vi "Framework Listener Sobot.vi"() -> ()   [LabVIEW 2017]
uses:
  TypeDefinitions/TCP Cluster.ctl
  TypeDefinitions/TCP Commands.ctl
  TypeDefinitions/Sobot Driving Data.ctl
  <vilib>/Utility/inputDevices.llb/closeJoystick.vi
  <vilib>/Instr/_visa.llb/VISA Configure Serial Port (Instr).vi
panel:
  out "value":T1
  out "Driving Data":u8[](array[numeric])
  in  "stop 2":bool
  in  "device index":i32
  in  "Manuelles Fahren (Joystick)":bool
  in  "VISA resource name":refnum<visa-resource-name>
  out "Send":T2={"Datatype"=enum."Message", "String"="Send to sobot"}
  out "Receive":T2={"Datatype"=enum."Message", "String"="Send to sobot"}
  in  "Button 2":bool
  in  "stop":bool
  in  "Button 1":bool
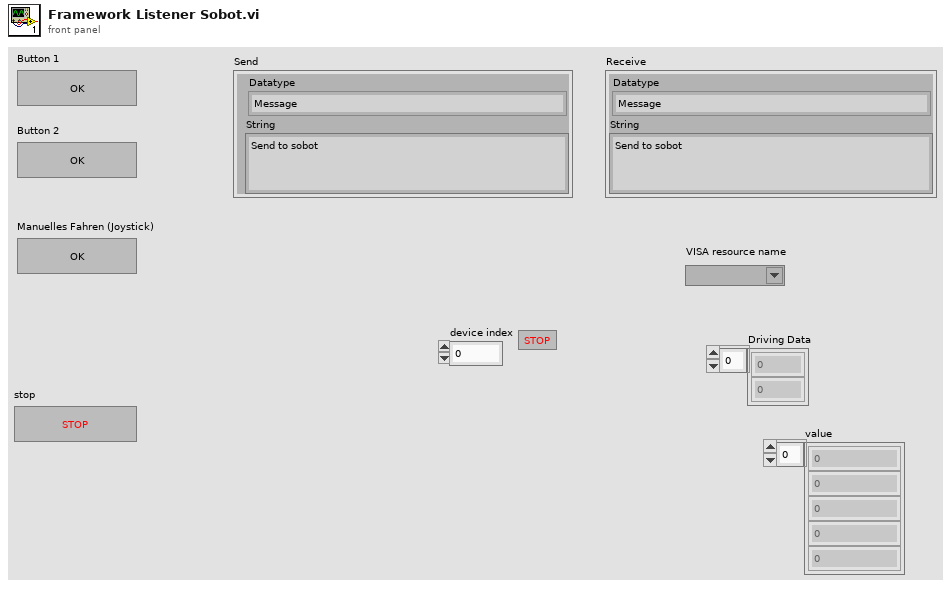
[diagram p1: front panel]
types:
  T1 = typedef "Sobot Driving Data.ctl" = u8[]
  T2 = typedef "TCP Cluster.ctl" = cluster{"Datatype":T3, "String":string}
  T3 = typedef "TCP Commands.ctl" = enum16{"Message", "sobotManualDrive", "Stop", "Command"}
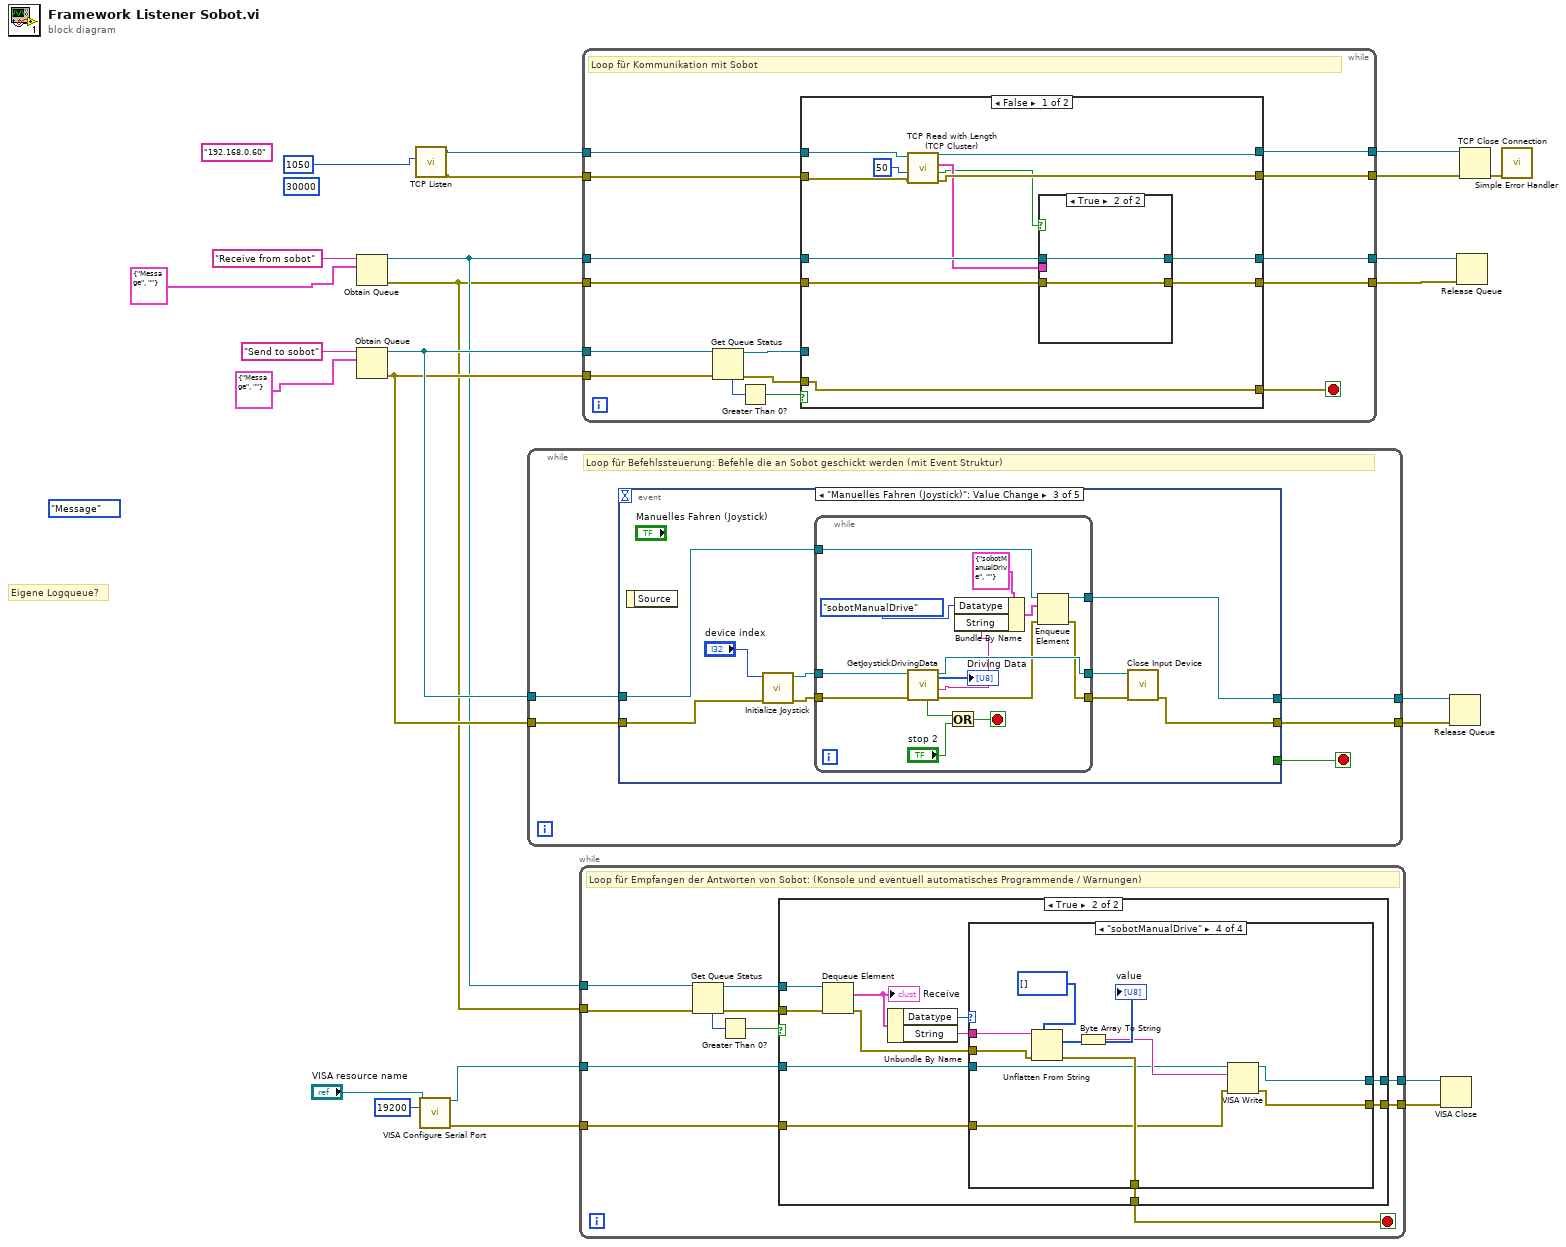
[diagram p0: block diagram]
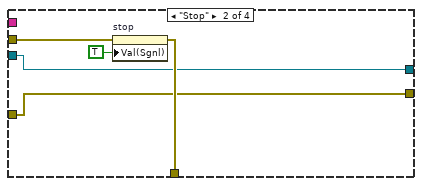
[diagram p4: hidden frame]
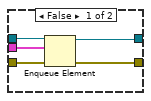
[diagram p6: hidden frame]
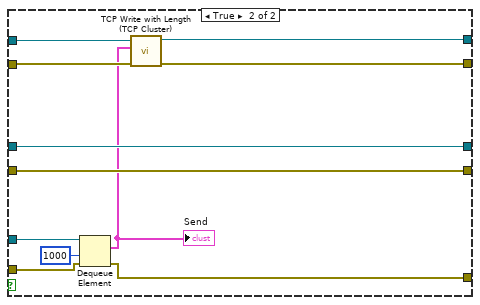
[diagram p7: hidden frame]
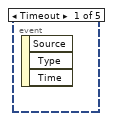
[diagram p8: hidden frame]
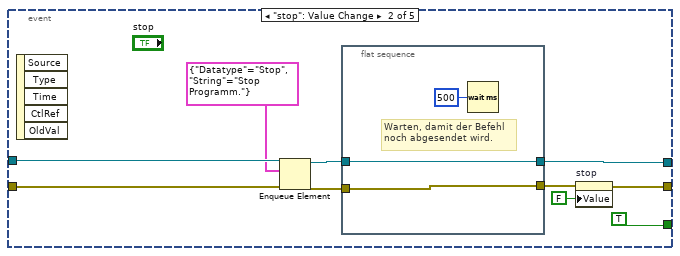
[diagram p9: hidden frame]
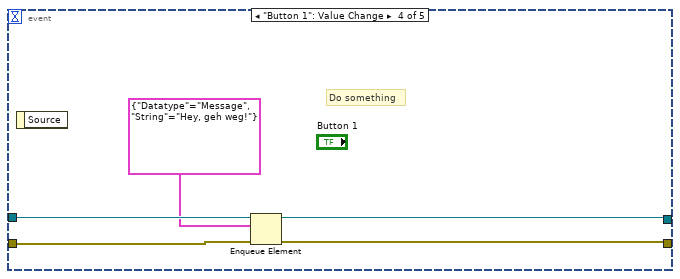
[diagram p10: hidden frame]
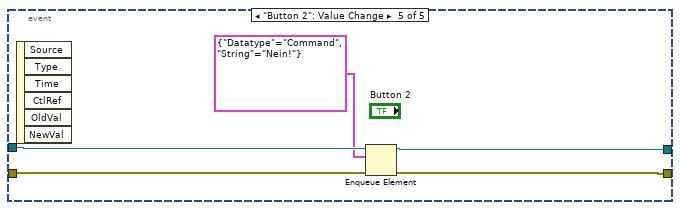
[diagram p11: hidden frame]
diagram:
  (unwired) TCP_Commands."Message"
  (unwired) 30000 ("timeout ms (60000)")
  (unwired) "192.168.0.60" ("address")
  # "Eigene Logqueue?"
  n1 = Obtain Queue(name (unnamed)="Receive from sobot", element data type=T2 {"Datatype"=enum."Message", "String"=""}) -> (queue out=w15:refnum<queue>, error out=w14:errorcluster)  [unwired: 3 in, 1 out]
  n2 = Obtain Queue(name (unnamed)="Send to sobot", element data type=T2 {"Datatype"=enum."Message", "String"=""}) -> (queue out=w23:refnum<queue>, error out=w20:errorcluster)  [unwired: 3 in, 1 out]
  n3 = call <vilib>:"TCP Listen.vi"("port"=u16 1050 ("remote port or service name")) -> ("error out"=w2:errorcluster, "connection ID"=w3:refnum<k5>)  [unwired: 6 in, 3 out]
  n4 = call-poly "VISA Configure Serial Port"("VISA resource name"="VISA resource name", "baud rate (9600)"=u32 19200) -> ("VISA resource name out"=w5:refnum<visa-resource-name>, "error out"=w4:errorcluster)  [unwired: 12 in]
  n5 = while {
    tunnel: w23 -> [w28]
    tunnel: [w27] -> w22
    tunnel: [w26] -> w21
    tunnel: w20 -> [w25]
    stop <- w29 stop-if-true
    # "Loop für Befehlssteuerung: Befehle die an Sobot geschickt werden (mit Event Struktur)"
    n6 = event shown="[2] \"Manuelles Fahren (Joystick)\": Value Change" {
      selector: _ -> [_ _ _ _ _]
      dyn-events: _ -> [_ _ _ _ _]
      timeout: _ -> [_ _ _ _ _]
      tunnel: [_ TRUE _ _ _] -> w29
      tunnel: w28 -> [_ w38 w44 w71 w76]
      tunnel: [_ w34 w43 w68 w75] -> w27
      tunnel: [_ w31 w45 w69 w74] -> w26
      tunnel: w25 -> [_ w37 w46 w70 w73]
      event Timeout {
        n7 = event-data() -> ()  [unwired: 1 in, 3 out]
      }
      event "stop": Value Change {
        n8 = event-data() -> ()  [unwired: 1 in, 5 out]
        n9 = Enqueue Element(queue=w38, element=T2 {"Datatype"=enum."Stop", "String"="Stop Programm."}, error in (no error)=w37) -> (queue out=w35:refnum<queue>, error out=w33:errorcluster)  [unwired: 1 in, 1 out]
        n10 = flat-sequence {
          tunnel: w35 -> [w42]
          tunnel: [w42] -> w34
          tunnel: [w40] -> w32
          tunnel: w33 -> [w40]
          frame #0 {
            # "Warten, damit der Befehl\nnoch abgesendet wird."
            n11 = Wait (ms)(milliseconds to wait=u32 500) -> ()  [unwired: 1 out]
          }
        }
        n12 = property on="stop" class="Bool (strict)"(error in=w32, "Value"=FALSE ("stop")) -> (error out=w31:errorcluster)  [unwired: 1 in, 1 out]
      }
      event "Manuelles Fahren (Joystick)": Value Change {
        n13 = event-data() -> ()  [unwired: 1 in, 1 out]
        n14 = call <vilib>:"Initialize Joystick.vi"("error in (no error)"=w46, "device index"="device index") -> ("error out"=w50:errorcluster, "device ID"=w51:refnum<k1>)  [unwired: 8 in]
        n15 = while {
          tunnel: w51 -> [w66]
          tunnel: w50 -> [w65]
          tunnel: [w64] -> w48
          tunnel: [w52] -> w47
          tunnel: w44 -> [w55]
          tunnel: [w54] -> w43
          stop <- w61 stop-if-true
          n16 = call "GetJoystickDrivingData.vi"("error in (no error)"=w65, "Refnum in"=w66) -> ("error out"=w53:errorcluster, "data string"=w58:string, "Refnum out"=w64:refnum<k1>, "Boolean"=w62:bool, "Array"=→"Driving Data":u8[])  [unwired: 4 in, 1 out]
          n17 = Or(x=w62, y="stop 2") -> (x .or. y?=w61:bool)
          n18 = Bundle By Name(cluster=T2 {"Datatype"=enum."sobotManualDrive", "String"=""}, "Datatype"=TCP_Commands."sobotManualDrive", "String"=w58) -> (w56:T2)
          n19 = Enqueue Element(queue=w55, element=w56, error in (no error)=w53) -> (queue out=w54:refnum<queue>, error out=w52:errorcluster)  [unwired: 1 in, 1 out]
        }
        n20 = call-poly <vilib>:"Close Input Device.vi"("error in (no error)"=w47, "device ID"=w48) -> ("error out"=w45:errorcluster)  [unwired: 8 in]
      }
      event "Button 1": Value Change {
        # "Do something"
        n21 = event-data() -> ()  [unwired: 1 in, 1 out]
        n22 = Enqueue Element(queue=w71, element=T2 {"Datatype"=enum."Message", "String"="Hey, geh weg!"}, error in (no error)=w70) -> (queue out=w68:refnum<queue>, error out=w69:errorcluster)  [unwired: 1 in, 1 out]
      }
      event "Button 2": Value Change {
        n23 = event-data() -> ()  [unwired: 1 in, 6 out]
        n24 = Enqueue Element(queue=w76, element=T2 {"Datatype"=enum."Command", "String"="Nein!"}, error in (no error)=w73) -> (queue out=w75:refnum<queue>, error out=w74:errorcluster)  [unwired: 1 in, 1 out]
      }
    }
  }
  n25 = while {
    tunnel: w15 -> [w86]
    tunnel: w14 -> [w85]
    tunnel: [w80] -> w9
    tunnel: [w79] -> w8
    tunnel: w5 -> [w78]
    tunnel: w4 -> [w77]
    stop <- w81 stop-if-true
    # "Loop für Empfangen der Antworten von Sobot: (Konsole und eventuell automatisches Programmende / Warnungen)"
    n26 = Get Queue Status(queue=w86, error in (no error)=w85) -> (queue out=w83:refnum<queue>, error out=w82:errorcluster, # elements in queue=w87:i32)  [unwired: 1 in, 5 out]
    n27 = Greater Than 0?(x=w87) -> (x > 0?=w84:bool)
    n28 = case shown="True" w84 {
      tunnel: w83 -> [_ w101]
      tunnel: w82 -> [w90 w100]
      tunnel: [w90 w96] -> w81
      tunnel: [w88 w94] -> w80
      tunnel: [w89 w93] -> w79
      tunnel: w78 -> [w89 w92]
      tunnel: w77 -> [w88 w91]
      frame False {
      }
      frame True {
        n29 = Dequeue Element(queue=w101, error in (no error)=w100) -> (element=w99:T2, error out=w97:errorcluster)  [unwired: 1 in, 2 out]
        "Receive" <- w99
        n30 = Unbundle By Name(w99) -> ("Datatype"=w98:T3, "String"=w95:string)
        n31 = case shown="\"sobotManualDrive\"" w98 {
          tunnel: w97 -> [w104 w108 w112 w120]
          tunnel: [w104 w107 w112 w119] -> w96
          tunnel: w95 -> [_ _ _ w122]
          tunnel: [w102 w105 w110 w116] -> w94
          tunnel: [w103 w106 w111 w115] -> w93
          tunnel: w92 -> [w103 w106 w111 w114]
          tunnel: w91 -> [w102 w105 w110 w113]
          frame "Message", Default {
          }
          frame "Stop" {
            n32 = property on="stop" class="Bool (strict)"(error in=w108, "Val(Sgnl)"=TRUE ("Value (Signaling)")) -> (error out=w107:errorcluster)  [unwired: 1 in, 1 out]
          }
          frame "Command" {
          }
          frame "sobotManualDrive" {
            n33 = Unflatten From String(type=T1 [] ("Sobot Driving Data"), binary string=w122, error in (no error)=w120) -> (value=w118:T1, error out=w119:errorcluster)  [unwired: 2 in, 1 out]
            "value" <- w118
            n34 = Byte Array To String(unsigned byte array=w118) -> (string=w117:string)
            n35 = VISA Write(VISA resource name=w114, write buffer=w117, error in (no error)=w113) -> (VISA resource name out=w115:refnum<visa-resource-name>, error out=w116:errorcluster)  [unwired: 1 out]
          }
        }
      }
    }
  }
  n36 = while {
    tunnel: w23 -> [w136]
    tunnel: w20 -> [w134]
    tunnel: w3 -> [w130]
    tunnel: w2 -> [w129]
    tunnel: [w128] -> w18
    tunnel: [w127] -> w17
    tunnel: w15 -> [w126]
    tunnel: w14 -> [w125]
    tunnel: [w124] -> w12
    tunnel: [w123] -> w13
    stop <- w137 stop-if-true
    # "Loop für Kommunikation mit Sobot"
    n37 = Get Queue Status(queue=w136, error in (no error)=w134) -> (queue out=w135:refnum<queue>, error out=w133:errorcluster, # elements in queue=w132:i32)  [unwired: 1 in, 5 out]
    n38 = Greater Than 0?(x=w132) -> (x > 0?=w131:bool)
    n39 = case shown="False" w131 {
      tunnel: [w149 w167] -> w137
      tunnel: w135 -> [_ w165]
      tunnel: w133 -> [w149 w164]
      tunnel: w130 -> [w144 w161]
      tunnel: w129 -> [w143 w160]
      tunnel: [w141 w159] -> w127
      tunnel: [w140 w158] -> w128
      tunnel: w126 -> [w148 w163]
      tunnel: w125 -> [w147 w162]
      tunnel: [w146 w163] -> w123
      tunnel: [w145 w162] -> w124
      frame False {
        n40 = call "TCP Read with Length (TCP Cluster).vi"("error in (no error)"=w143, "Timeout"=50, "connection ID"=w144) -> ("error out"=w141:errorcluster, "Timeout?"=w138:bool, "TCP Cluster"=w139:T2, "connection ID out"=w140:refnum<k5>)  [unwired: 5 in]
        n41 = case shown="True" w138 {
          tunnel: w148 -> [w154 w156]
          tunnel: w147 -> [w153 w155]
          tunnel: w139 -> [w152 _]
          tunnel: [w151 w156] -> w146
          tunnel: [w150 w155] -> w145
          frame False {
            n42 = Enqueue Element(queue=w154, element=w152, error in (no error)=w153) -> (queue out=w151:refnum<queue>, error out=w150:errorcluster)  [unwired: 1 in, 1 out]
          }
          frame True {
          }
        }
      }
      frame True {
        n43 = Dequeue Element(queue=w165, timeout in ms (-1)=1000, error in (no error)=w164) -> (element=w157:T2, error out=w167:errorcluster)  [unwired: 2 out]
        "Send" <- w157
        n44 = call "TCP Write with Length (TCP Cluster).vi"("error in (no error)"=w160, 10:w157, "connection ID"=w161) -> ("error out"=w159:errorcluster, "connection ID out"=w158:refnum<k5>)  [unwired: 7 in]
      }
    }
  }
  n45 = VISA Close(VISA resource name=w8, error in (no error)=w9) -> ()  [unwired: 1 out]
  n46 = Release Queue(queue=w22, error in (no error)=w21) -> ()  [unwired: 1 in, 3 out]
  n47 = Release Queue(queue=w13, error in (no error)=w12) -> ()  [unwired: 1 in, 3 out]
  n48 = TCP Close Connection(connection ID=w18, error in (no error)=w17) -> (error out=w19:errorcluster)  [unwired: 1 in, 1 out]
  n49 = call <vilib>:"Simple Error Handler.vi"("error in (no error)"=w19) -> ()  [unwired: 4 in, 5 out]
